vi "LeCroy Wave Series Transfer Selected Waveform.vi"() -> ()   [LabVIEW 2018]
doc: "This example shows how to readback data using the Fetch Waveform vi. No changes are made to the instrument's configuration, making this a very easy example to use. \n\nDirections:\n1. Configure the scope manually and execute a SINGLE trigger to get a waveform on the desired channel.\n\n2. On this front panel, enter the VISA Resource name for your scope. (e.g VICP:123.45.67.8 for TCP/IP, GPIB::5::INSTR for GPIB)\n\n3. Select your source and modify your timeout if necessary (10000ms should be more than sufficient)\n\n4. Run the VI to readback the data."
uses:
  LeCroy Wave Series.lvlib
panel:
  in  "Source (0: Channel 1)":u16(ring) items=["Channel 1", "Channel 2", "Channel 3", "Channel 4", "Memory 1", "Memory 2", "Memory 3", "Memory 4", "Function 1", "Function 2", "Function 3", "Function 4", "Function 5", "Function 6", "Function 7", "Function 8"]
  in  "Timeout (10000 ms)":u32=10000
  out "Waveform Data":waveform(dbl)(graph)
  in  "VISA resource name":refnum<visa-resource-name>
  # "(c) 2008 - 2012 NATIONAL INSTRUMENTS.  ALL RIGHTS RESERVED."
  # "Directions:\n\n1. Configure the scope manually and execute a SINGLE trigger to get a waveform on the desired channel.\n\n2. On this front panel, enter the VISA Resource name for your scope. (e.g VICP::123.45.67.8 for TCP/IP, GPIB::5::INSTR for GPIB)\n\n3. Select your source and modify your timeout if necessary (10000ms should be more than sufficient)\n\n4. Run the VI to readback the data."
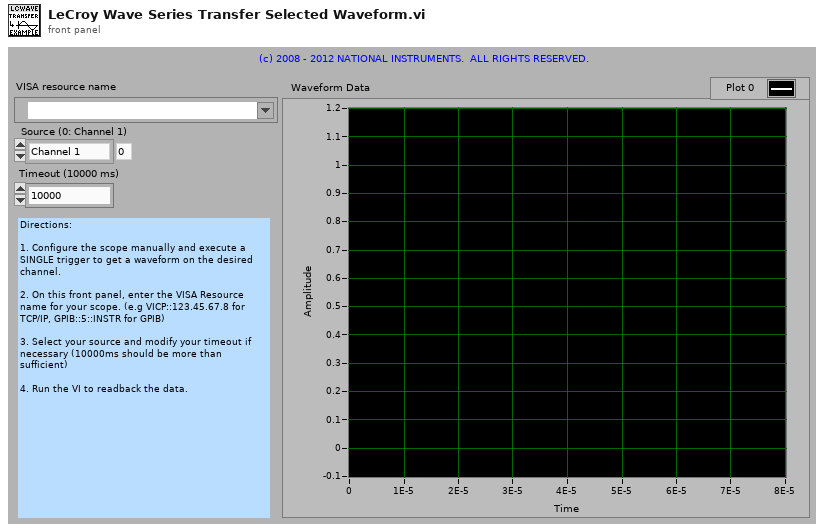
[diagram p1: front panel]
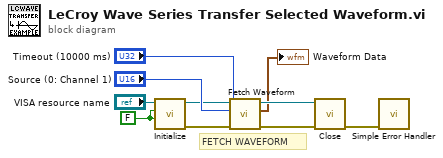
[diagram p0: block diagram]
diagram:
  w1 = FALSE ("Reset? (T: Yes)")
  # "FETCH WAVEFORM"
  n1 = call "Initialize.vi"("Reset? (T: Yes)"=w1, "ID Query? (T: Yes)"=w1, "VISA resource name"="VISA resource name") -> ("error out"=w3:errorcluster, "VISA resource name out"=w2:refnum<visa-resource-name>)  [unwired: 7 in]
  n2 = call "Fetch Waveform.vi"("error in (no error)"=w3, "Timeout (10000 ms)"="Timeout (10000 ms)", "Source (0: Channel 1)"="Source (0: Channel 1)", "VISA resource name"=w2) -> ("error out"=w8:errorcluster, "Waveform Graph"=→"Waveform Data":waveform(dbl), "VISA resource name out"=w9:refnum<visa-resource-name>)  [unwired: 5 in]
  n3 = call "Close.vi"("error in (no error)"=w8, "VISA resource name"=w9) -> ("error out"=w10:errorcluster)  [unwired: 9 in]
  n4 = call <vilib>:"Simple Error Handler.vi"("error in (no error)"=w10) -> ()  [unwired: 4 in, 5 out]
